vi "Configure Trigger Model Blender Mode.vi"(8 "error in (no error)":errorcluster, 9 "Orenable Mode (AND)":u16(ring) items=["AND", "OR"], 10 "Blender Number (1-2)":i32=1 min=1 max=2 step=1 format="%#.6g", 11 "VISA resource name":refnum<visa-resource-name>) -> (0 "error out":errorcluster, 3 "VISA resource name out":refnum<visa-resource-name>)   [LabVIEW 2017, in "Keithley 2450.lvlib"]
doc: "This VI selects whether the blender performs OR operations or AND operations."
uses:
  Keithley 2450.lvlib
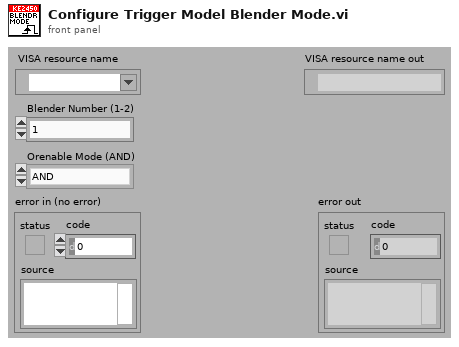
[diagram p1: front panel]
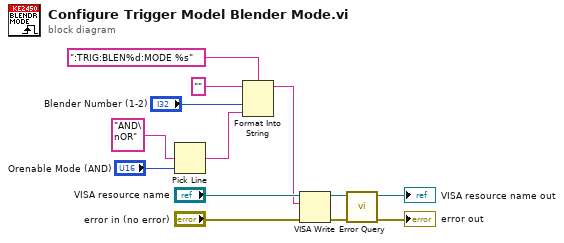
[diagram p0: block diagram]
diagram:
  n1 = Pick Line(multi-line string="AND\nOR", line index="Orenable Mode (AND)") -> (output string=w1:string)  [unwired: 1 in]
  n2 = Format Into String(format string=":TRIG:BLEN%d:MODE %s", initial string="", "Blender Number (1-2)", w1) -> (resulting string=w4:string)  [unwired: 1 in, 1 out]
  n3 = VISA Write(VISA resource name="VISA resource name", write buffer=w4, error in (no error)="error in (no error)") -> (VISA resource name out=w9:refnum<visa-resource-name>, error out=w8:errorcluster)  [unwired: 1 out]
  n4 = call "Error Query.vi"("error in (no error)"=w8, "VISA resource name"=w9) -> ("error out"=→"error out":errorcluster, "VISA resource name out"=→"VISA resource name out":refnum<visa-resource-name>)  [unwired: 8 out]
